vi "dll.midi_get_output_device_count.vi"(8 "error in (no error)":errorcluster, 11 "midi out in":refnum<class "midi out.lvclass">) -> (0 "error out":errorcluster, 2 "Device Count":i32, 3 "midi out":refnum<class "midi out.lvclass">)   [LabVIEW 2020, in "midi out.lvclass"]
uses:
  midi out.lvclass
  midi out.lvclass/midi out.ctl
  shared/midi shared.lvlib
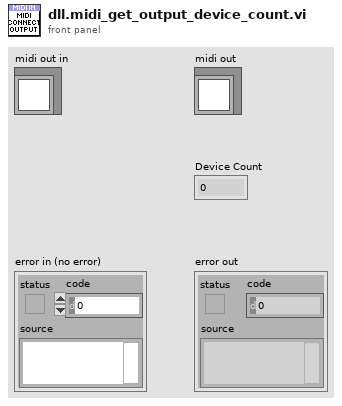
[diagram p1: front panel]
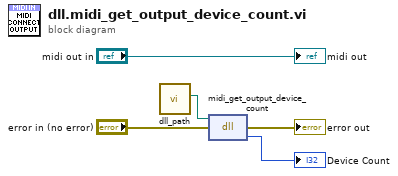
[diagram p0: block diagram]
diagram:
  n1 = call "dll_path.vi"() -> ("dll"=w4:path)  [unwired: 11 in]
  n2 = dll-call lib="C:/code/LabVIEW-MIDI-XPLAT/dist/TomMIDIllan_*.*" fn="midi_get_output_device_count"(path in=w4, error in="error in (no error)") -> (error out=→"error out":errorcluster, "Device Count"=→"Device Count":i32)  [unwired: 1 in, 1 out]
  "midi out" <- "midi out in"
